vi "Query Correction Table Entries.vi"(8 "error in (no error)":errorcluster, 10 "Correction Table (\"Table1\")":string="Table1", 11 "VISA resource name":refnum<visa-resource-name>) -> (0 "error out":errorcluster, 2 "Entries":cluster{"Frequency":dbl, "Attenuation":dbl}[](array[cluster]) {"Attenuation" format="%#_6f"; "Frequency" format="%#_6e"}, 3 "VISA resource name out":refnum<visa-resource-name>)   [LabVIEW 2015, in "Rohde&Schwarz CMXP Base.lvlib"]
doc: "Returns the entries of a correction table.\n\nAttribute:\n-\n\nRemote-control command:\n[CONFigure:]SYSTem:ATTenuation:CTABle:INFO?"
uses:
  <instrlib>/Rohde&Schwarz CMXP Base/Rohde&Schwarz CMXP Base.lvlib
  <instrlib>/Rohde&Schwarz CMXP Base/Private/rsidr_core.llb/rsidr_core.lvlib
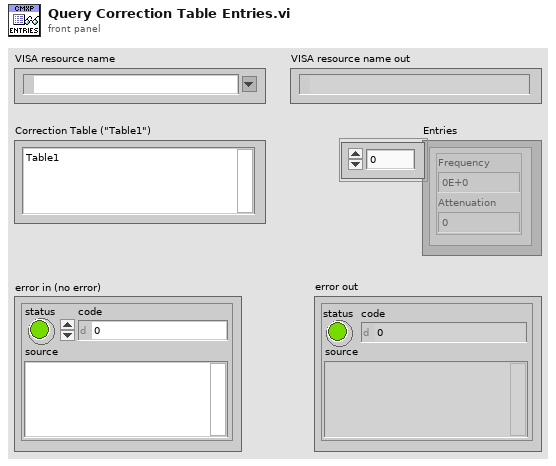
[diagram p1: front panel]
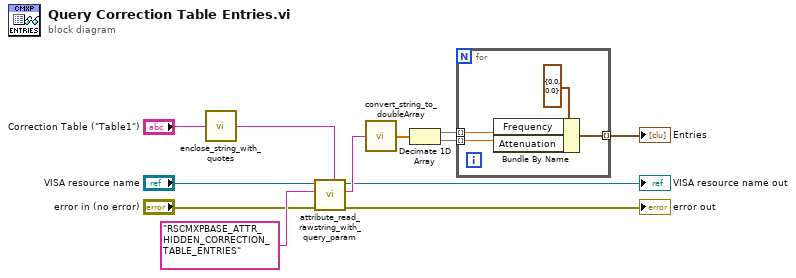
[diagram p0: block diagram]
diagram:
  n1 = call <instrlib>:"enclose_string_with_quotes.vi"("String to enclose"="Correction Table (\"Table1\")") -> ("String out"=w1:string)  [unwired: 4 in]
  n2 = call <instrlib>:"attribute_read_rawstring_with_query_param.vi"("Query Parameter (None)"=w1, "error in"="error in (no error)", "Attribute ID"="RSCMXPBASE_ATTR_HIDDEN_CORRECTION_TABLE_ENTRIES", "VISA resource name"="VISA resource name") -> ("error out"=→"error out":errorcluster, "RawString out"=w11:string, "VISA resource name out"=→"VISA resource name out":refnum<visa-resource-name>)  [unwired: 5 in]
  n3 = call <instrlib>:"convert_string_to_doubleArray.vi"("string in"=w11) -> ("double array out"=w10:dbl[])  [unwired: 3 in, 1 out]
  n4 = Decimate 1D Array(w10) -> (w9:dbl[], w8:dbl[])
  n5 = for {
    tunnel: w9 -> [w15] mode=indexing
    tunnel: w8 -> [w14] mode=indexing
    tunnel: [w13] -> w7 mode=indexing
    n6 = Bundle By Name(cluster=cluster{"Frequency":dbl, "Attenuation":dbl} {"Frequency"=0.0, "Attenuation"=0.0} ("Entry"), "Frequency"=w15, "Attenuation"=w14) -> (w13:cluster{"Frequency":dbl, "Attenuation":dbl})
  }
  "Entries" <- w7
